vi "FlatToRichni_measurementlink_pinmap_v1_QueryPinsResponse.vi"(5 "OutputClusterType":T1, 11 "InputCluster":T4) -> (3 "OutputCluster":T1)   [LabVIEW 2021, in "ni.measurementlink.pinmap.v1.api.lvlib"]
uses:
  ni.measurementlink.pinmap.v1.api.lvlib
  ni_measurementlink_pinmap_v1_QueryPinsResponse_Flat.ctl
  ni_measurementlink_pinmap_v1_PinDefinition_Flat.ctl
  ni_measurementlink_pinmap_v1_PinGroupDefinition_Flat.ctl
  ni_measurementlink_pinmap_v1_QueryPinsResponse.ctl
  ni_measurementlink_pinmap_v1_PinDefinition.ctl
  ni_measurementlink_pinmap_v1_PinGroupDefinition.ctl
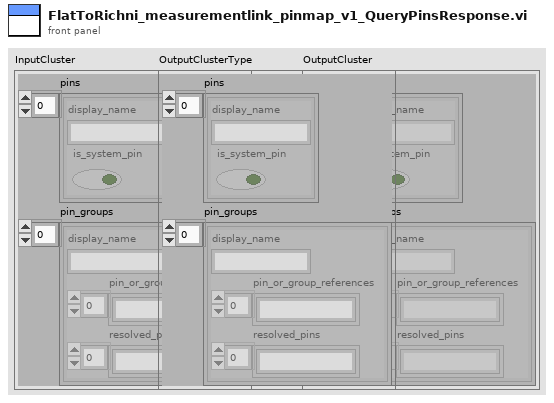
[diagram p1: front panel]
types:
  T1 = typedef "ni.measurementlink.pinmap.v1.api.lvlib/ni_measurementlink_pinmap_v1_QueryPinsResponse.ctl" = cluster{"pins":T2[], "pin_groups":T3[]}
  T2 = typedef "ni.measurementlink.pinmap.v1.api.lvlib/ni_measurementlink_pinmap_v1_PinDefinition.ctl" = cluster{"display_name":string, "is_system_pin":bool}
  T3 = typedef "ni.measurementlink.pinmap.v1.api.lvlib/ni_measurementlink_pinmap_v1_PinGroupDefinition.ctl" = cluster{"display_name":string, "pin_or_group_references":string[], "resolved_pins":string[]}
  T4 = typedef "ni.measurementlink.pinmap.v1.api.lvlib/ni_measurementlink_pinmap_v1_QueryPinsResponse_Flat.ctl" = cluster{"pins":T5[], "pin_groups":T6[]}
  T5 = typedef "ni.measurementlink.pinmap.v1.api.lvlib/ni_measurementlink_pinmap_v1_PinDefinition_Flat.ctl" = cluster{"display_name":string, "is_system_pin":bool}
  T6 = typedef "ni.measurementlink.pinmap.v1.api.lvlib/ni_measurementlink_pinmap_v1_PinGroupDefinition_Flat.ctl" = cluster{"display_name":string, "pin_or_group_references":string[], "resolved_pins":string[]}
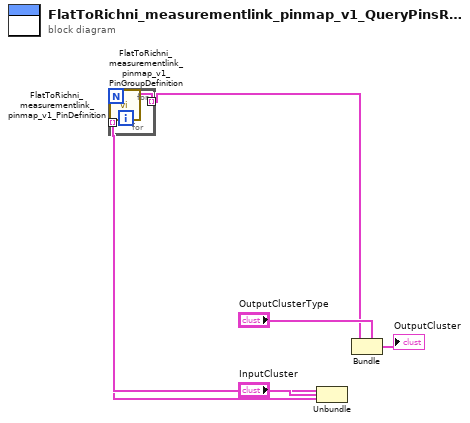
[diagram p0: block diagram]
diagram:
  n1 = Unbundle "Unbundle"("InputCluster") -> ("pins"=w4:T5[], "pin_groups"=w2:T6[])
  n2 = for {
    tunnel: w2 -> [w9] mode=indexing
    tunnel: [w8] -> w1 mode=indexing
    n3 = call "FlatToRichni_measurementlink_pinmap_v1_PinGroupDefinition.vi"("InputCluster"=w9) -> ("OutputCluster"=w8:T3)  [unwired: 10 in]
  }
  n4 = for {
    tunnel: w4 -> [w11] mode=indexing
    tunnel: [w10] -> w3 mode=indexing
    n5 = call "FlatToRichni_measurementlink_pinmap_v1_PinDefinition.vi"("InputCluster"=w11) -> ("OutputCluster"=w10:T2)  [unwired: 10 in]
  }
  n6 = Bundle "Bundle"(cluster="OutputClusterType", "pins"=w3, "pin_groups"=w1) -> (→"OutputCluster":T1)
